vi "sendValue.vi"(8 "error in (no error)":errorcluster, 10 "data":variant, 11 "stopMotionAllAxis in":refnum<class "stopMotionAllAxis.lvclass">) -> (0 "error out":errorcluster, 2 "function return":i32, 3 "stopMotionAllAxis out":refnum<class "stopMotionAllAxis.lvclass">)   [LabVIEW 2016, in "SALLV_AtDome_Messaging.lvlib" / "stopMotionAllAxis.lvclass"]
uses:
  stopMotionAllAxis.lvclass
  ts_sallv_AtDome/DataTypes/command_stopAzimuth.ctl
  ts_sallv_AtDome/SALLV_AtDome.lvlib
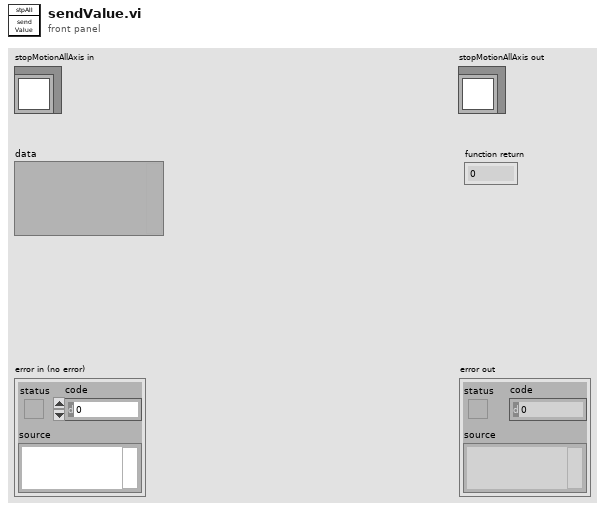
[diagram p1: front panel]
types:
  T1 = typedef "SALLV_AtDome.lvlib/command_stopAzimuth.ctl" = cluster{"value":bool}
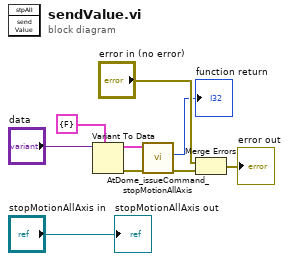
[diagram p0: block diagram]
diagram:
  n1 = Variant To Data(type=T1 {"value"=FALSE} ("data"), Variant="data") -> (data=w3:T1, error out=w4:errorcluster)  [unwired: 1 in]
  n2 = call "AtDome_issueCommand_stopMotionAllAxis.vi"("error in (no error)"=w4, "command_stopMotionAllAxis_Ctl"=w3) -> ("error out"=w1:errorcluster, "function return"=→"function return":i32)  [unwired: 7 in, 1 out]
  n3 = Merge Errors("error in (no error)", w1) -> (→"error out":errorcluster)
  "stopMotionAllAxis out" <- "stopMotionAllAxis in"
